vi "Get initialization status.vi"(8 "error in (no error)":errorcluster, 11 "RxTx in":refnum<class "RxTx.lvclass">) -> (0 "error out":errorcluster, 3 "RxTx out":refnum<class "RxTx.lvclass">)   [LabVIEW 2018, in "RxTx.lvclass"]
uses:
  RxTx.lvclass
  RxTx.lvclass/RxTx.ctl
  Interface/Interface.lvclass
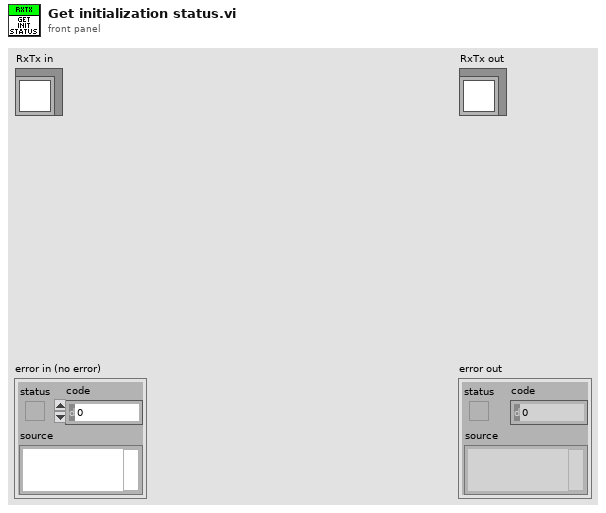
[diagram p1: front panel]
types:
  T1 = cluster{"Initialization":bool, "Serial Number":u16}
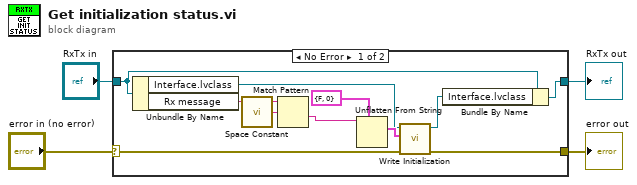
[diagram p0: block diagram]
diagram:
  n1 = case shown="No Error" "error in (no error)" {
    selector: "error in (no error)" -> [w9 w17]
    tunnel: [w8 w17] -> w3
    tunnel: [w5 w16] -> w1
    tunnel: "RxTx in" -> [w7 w16]
    frame No Error {
      n2 = Unbundle By Name(w7) -> ("Interface.lvclass"=w10:refnum<class "Interface.lvclass">, "Rx message"=w15:string)
      n3 = call <vilib>:"Space Constant.vi"() -> ("String"=w14:string)
      n4 = Match Pattern(string=w15, regular expression=w14) -> (after substring=w13:string)  [unwired: 1 in, 3 out]
      n5 = Unflatten From String(type=T1 {"Initialization"=FALSE, "Serial Number"=0} ("Initialization"), binary string=w13) -> (value=w11:T1)  [unwired: 3 in, 2 out]
      n6 = call "Write Initialization.vi"("error in (no error)"=w9, "Initialization"=w11, "Interface in"=w10) -> ("error out"=w8:errorcluster, "Interface out"=w6:refnum<class "Interface.lvclass">)  [unwired: 7 in]
      n7 = Bundle By Name(cluster=w7, "Interface.lvclass"=w6) -> (w5:refnum<class "RxTx.lvclass">)
    }
    frame Error {
    }
  }
  "error out" <- w3
  "RxTx out" <- w1
